vi "ZMC Up Cur Zpj To Mem.vi"(7 "puifilesize":u32, 8 "error in (no error)":errorcluster caption="错误输入（无错误）", 9 "buffsize":u32, 10 "pbuffer":string, 11 "handle":u32) -> (0 "error out":errorcluster caption="错误输出", 1 "function return":i32, 2 "pbuffer out":string, 3 "handle out":u32, 5 "puifilesize out":u32)   [LabVIEW 2015, in "zauxdll.lvlib"]
doc: "int32 __stdcall ZMC_UpCurZpjToMem(ZMC_HANDLE handle, char* pbuffer, uint32 buffsize, uint32* puifilesize);"
uses:
  zauxdll.lvlib
  zmotion.dll
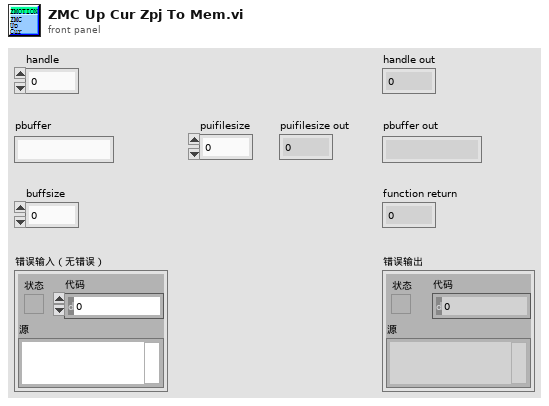
[diagram p1: front panel]
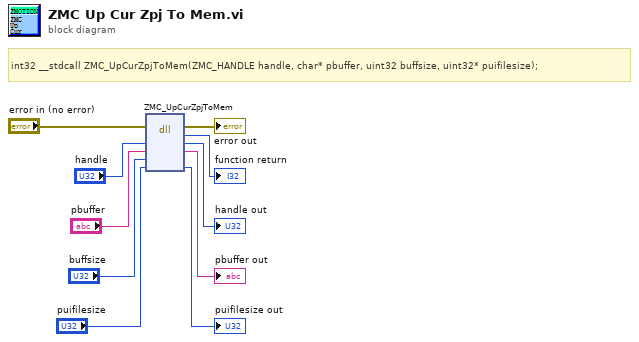
[diagram p0: block diagram]
diagram:
  # "int32 __stdcall ZMC_UpCurZpjToMem(ZMC_HANDLE handle, char* pbuffer, uint32 buffsize, uint32* puifilesize);"
  n1 = dll-call lib="C:/Users/VIC/Desktop/GOGORO_SA/system/LLB/zmotion/zaux/zmotion.*" fn="ZMC_UpCurZpjToMem"(error in="error in (no error)", "handle"="handle", "pbuffer"="pbuffer", "buffsize"="buffsize", "puifilesize"="puifilesize") -> (error out=→"error out":errorcluster, →"function return":i32, "handle"=→"handle out":u32, "pbuffer"=→"pbuffer out":string, "puifilesize"=→"puifilesize out":u32)  [unwired: 3 in, 1 out]
